vi "VerifyDeviceEnumDataIs.vi"(8 "error in":errorcluster) -> (0 "error out":errorcluster, 2 "DeviceID":i32, 3 "return value":i32)   [LabVIEW 2015]
doc: "Input Parameters:\n\n2: M4\n4: M5"
uses:
  ScannerDiagDLL.dll
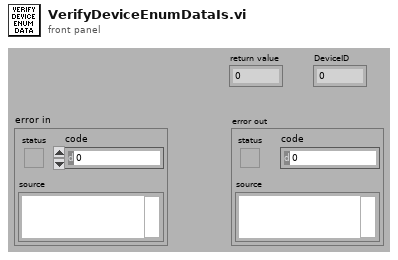
[diagram p1: front panel]
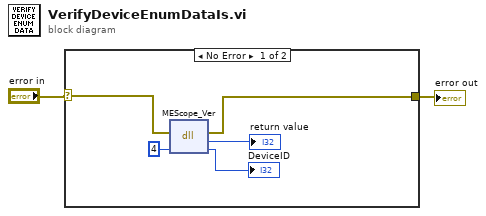
[diagram p0: block diagram]
diagram:
  n1 = case shown="No Error" "error in" {
    selector: "error in" -> [w5 w8]
    tunnel: [w4 w8] -> w1
    frame No Error {
      n2 = dll-call lib="C:/SNAPON/ModisEdge/TabletScope/Test Sequence/Code Modules/DLL/ScannerDiagDLL.dll" fn="MEScope_Ver"(error in=w5, "DeviceModelId"=4 ("arg1")) -> (error out=w4:errorcluster, "return type"=→"return value":i32, "DeviceModelId"=→"DeviceID":i32)  [unwired: 2 in, 1 out]
    }
    frame Error {
    }
  }
  "error out" <- w1
